vi "svc_Check for Waveform Parameter Continuity (1 Ch).vi"(7 "restart averaging (F)":bool, 8 "error in (no error)":errorcluster, 10 "checks for channel parameter change":T4, 11 "scaled signal [EU]":waveform(dbl)) -> (0 "error out":errorcluster, 1 "channel info":T1={"sensor sensitivity"=1000.0, "engineering units"=1, "dB reference"=1.0, "custom label"="EU", "weighting filter"=0, "pregain"=0.0} {"pregain" format="%.2f"; "weighting filter" items=["Linear", "A-weighting", "B-weighting", "C-weighting", "ITU-R 468-4", "Dolby", "CCITT", "C-message", "Wb", "Wc", "Wd", "We", "Wf", "Wh", "Wj", "Wk", "Wm", "AES17 20 kHz lowpass", "AES17 40 kHz lowpass", "AES17 20 kHz highpass", "AES17 40 kHz highpass"]; "dB reference" format="%^.1e"; "engineering units" items=["custom..."=0, "V"=1, "A"=21, "C"=30, "pC"=31, "s"=32, "-"=29, "Pa"=2, "N"=20, "g"=3, "m/s^2"=4, "m/s"=5, "m"=6, "mm/s"=12, "mm"=13, "micron/s"=14, "micron"=15, "in/s^2"=7, "in/s"=8, "in"=9, "mil/s"=10, "mil"=11, "rad/s^2"=16, "rad/s"=17, "rad"=18, "deg/s^2"=26, "deg/s"=27, "deg"=28, "RPM"=22, "cycle/s^2"=23, "Hz"=24, "cycle"=25, "strain"=19]; "sensor sensitivity" format="%#_5f"}, 2 "waveform parameter changed":bool, 3 "dup scaled signal [EU]":waveform(dbl), 4 "array length":i32, 5 "dt":dbl)   [LabVIEW 2017]
uses:
  <vilib>/addons/_NISVFA/_Shared subVIs/Controls/svc_Channel Info.ctl
  <vilib>/addons/_NISVFA/_Shared subVIs/Controls/svc_Engineering Units Text Ring.ctl
  <vilib>/addons/_NISVFA/_Shared subVIs/Controls/svc_Weighting Filter Text Ring.ctl
  <vilib>/addons/_NISVFA/_Shared subVIs/Common/svc_Get SV Channel Info.vi
  <vilib>/addons/_NISVFA/_Shared subVIs/Common/svc_Engineering Units to Unit Label.vi
  <vilib>/addons/_NISVFA/_Shared subVIs/Common/svc_Unit Label to Engineering Units.vi
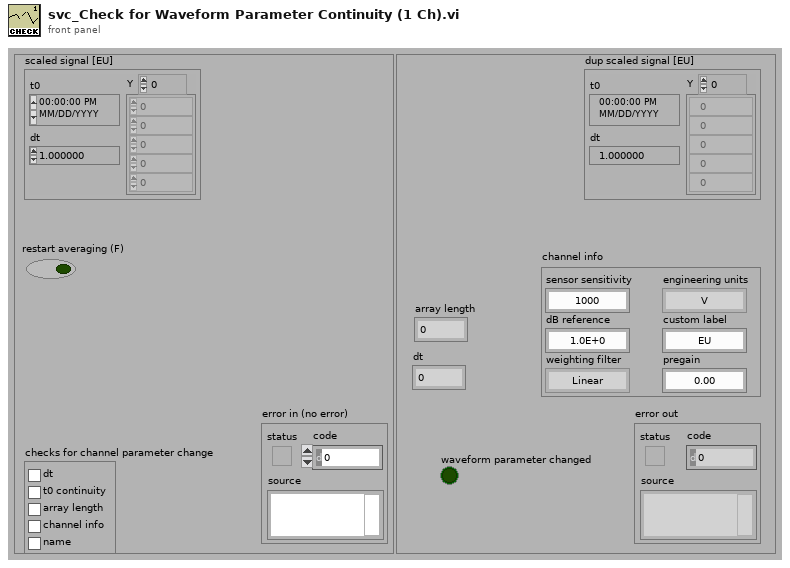
[diagram p1: front panel]
types:
  T1 = typedef "svc_Channel Info.ctl" = cluster{"sensor sensitivity":dbl, "engineering units":T2, "dB reference":dbl, "custom label":string, "weighting filter":T3, "pregain":dbl}
  T2 = typedef "svc_Engineering Units Text Ring.ctl" = u16
  T3 = typedef "svc_Weighting Filter Text Ring.ctl" = u16
  T4 = cluster{"dt":bool, "t0 continuity":bool, "array length":bool, "channel info":bool, "name":bool}
  T5 = typedef "svc_Waveform Parameters.ctl" = cluster{"channel name":string, "t0":timestamp, "dt":dbl, "array length":i32}
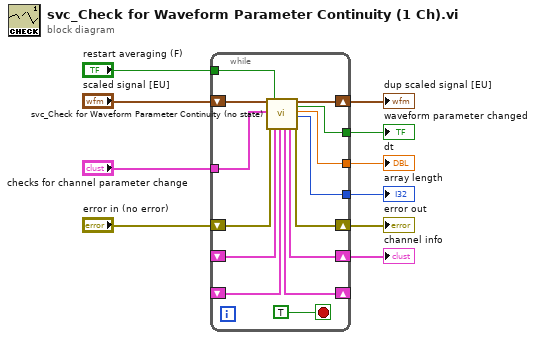
[diagram p0: block diagram]
diagram:
  n1 = while {
    tunnel: "checks for channel parameter change" -> [w15]
    tunnel: [w24] -> w7
    shift-right: [w21] -> _
    shift-left: _ -> [w20]
    tunnel: "restart averaging (F)" -> [w18]
    shift-right: [w17] -> w3
    shift-left: _ -> [w16]
    tunnel: [w12] -> w2
    tunnel: [w11] -> w1
    shift-right: [w13] -> w4
    shift-left: "scaled signal [EU]" -> [w23]
    shift-right: [w14] -> w9
    shift-left: "error in (no error)" -> [w19]
    stop <- TRUE stop-if-true
    n2 = call <vilib>:"svc_Check for Waveform Parameter Continuity (no state).vi"("scaled signal [EU]"=w23, "checks for channel parameter change"=w15, "error in (no error)"=w19, "reset"=w18, "expected channel info"=w16, "expected waveform parameters"=w20) -> ("next expected waveform parameters"=w21:T5, "next expected channel info"=w17:T1, "dup scaled signal [EU]"=w13:waveform(dbl), "waveform parameter changed"=w24:bool, "dt"=w12:dbl, "array length"=w11:i32, "error out"=w14:errorcluster)  [unwired: 7 in]
  }
  "error out" <- w9
  "waveform parameter changed" <- w7
  "dup scaled signal [EU]" <- w4
  "channel info" <- w3
  "dt" <- w2
  "array length" <- w1
